vi "Pre-chirper control L1.vi"(7 "State":enum16{"Initialise", "Query", "Close"}(ring), 8 "error in (no error)":errorcluster, 9 "Data to Set":dbl, 10 "Pre-chirper commands":T2, 11 "Visa resource":T1) -> (0 "error out":errorcluster, 3 "number":dbl)   [LabVIEW 2020]
uses:
  Prechirper commands.ctl
  Serial Comms/Visa resource.ctl
  Serial Comms/Serial - Settings.ctl
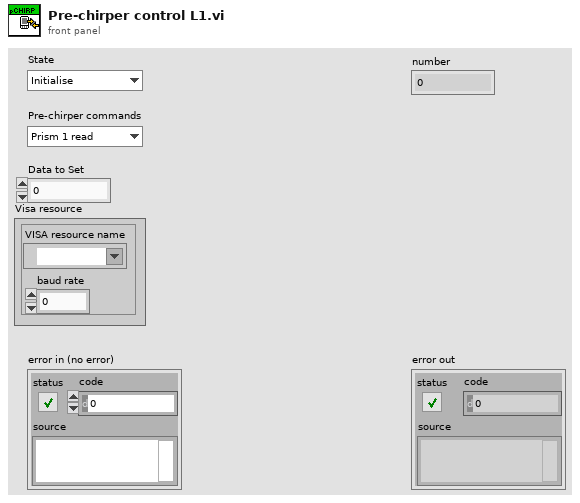
[diagram p1: front panel]
types:
  T1 = typedef "Visa resource.ctl" = cluster{"VISA resource name":refnum<visa-resource-name>, "baud rate":u32}
  T2 = typedef "Prechirper commands.ctl" = enum16{"Prism 1 read", "Prism 1 set", "Prism 2 read", "Prism 2 set", "Wavelength read", "Wavelength Femto set", "Wavelength Femto and Laser set", "GVD curve number read", "GVD curve number set"}
  T3 = typedef "Serial - Settings.ctl" = cluster{"VISA resource name ":refnum<visa-resource-name>, "baud rate":u32, "data bits":u16, "parity":enum16{"None", "Odd", "Even", "Mark", "Space"}, "stop bits":u16, "flow control":u16}
  T4 = enum16{"Initialise", "Read Handle", "Command & Query", "Close"}
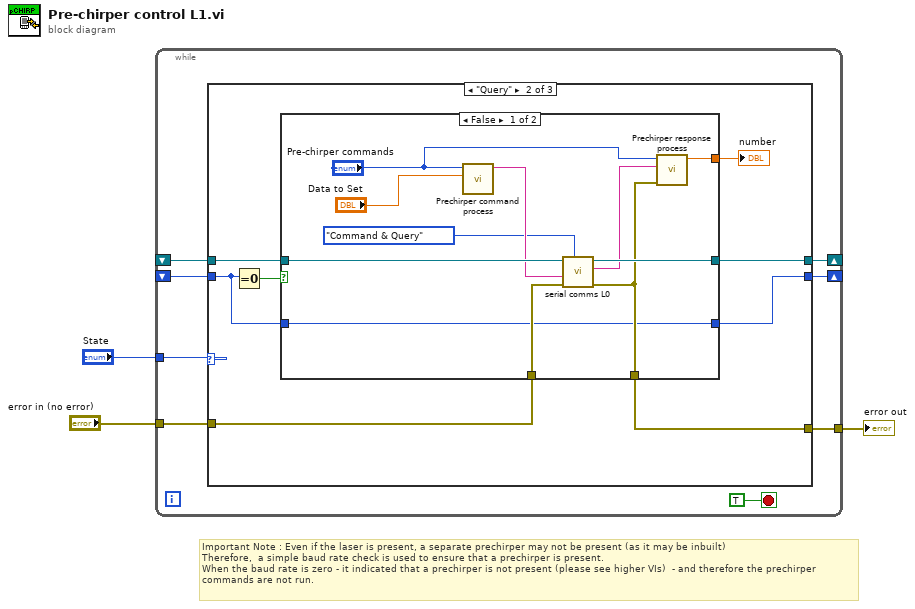
[diagram p0: block diagram]
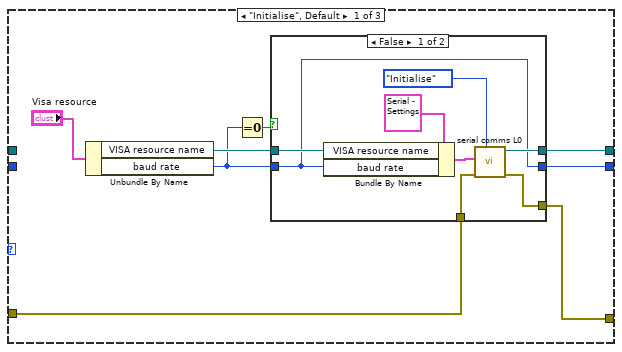
[diagram p2: hidden frame]
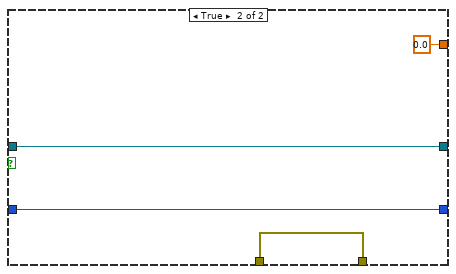
[diagram p4: hidden frame]
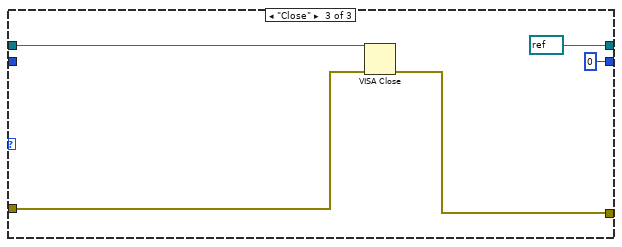
[diagram p5: hidden frame]
diagram:
  # "Important Note : Even if the laser is present, a separate prechirper may not be present (as it may be inbuilt)\nTherefore,  a simple baud rate check is used to ensure that a prechirper is present.\nWhen the baud rate is zero - it indicated that a prechirper is not present (please see higher VIs)  - and therefore the prechirper\ncommands are not run."
  n1 = while {
    tunnel: "State" -> [w10]
    tunnel: "error in (no error)" -> [w9]
    tunnel: [w8] -> w1
    shift-right: [w7] -> _
    shift-left: _ -> [w6]
    shift-right: [w5] -> _
    shift-left: _ -> [w4]
    stop <- TRUE stop-if-true
    n2 = case shown="\"Query\"" w10 {
      tunnel: w9 -> [w19 w38 w57]
      tunnel: [w18 w35 w56] -> w8
      tunnel: [w17 w36 refnum<visa-resource-name> refnum ("VISA resource name out")] -> w7
      tunnel: w6 -> [_ w37 w58]
      tunnel: [w12 w31 u32 0 ("baud rate")] -> w5
      tunnel: w4 -> [_ w32 _]
      frame "Initialise", Default {
        n3 = Unbundle By Name("Visa resource") -> ("VISA resource name"=w15:refnum<visa-resource-name>, "baud rate"=w14:u32)
        n4 = Equal To 0?(x=w14) -> (x = 0?=w13:bool)
        n5 = case shown="False" w13 {
          tunnel: w19 -> [w27 w29]
          tunnel: [w26 w29] -> w18
          tunnel: [w25 w30] -> w17
          tunnel: w15 -> [w22 w30]
          tunnel: w14 -> [w20 w28]
          tunnel: [w20 w28] -> w12
          frame False {
            n6 = Bundle By Name(cluster=T3 {"VISA resource name "="COM12", "baud rate"=115200, "data bits"=8, "parity"=enum."None", "stop bits"=10, "flow control"=0} ("Serial Settings"), "VISA resource name"=w22, "baud rate"=w20) -> (w21:T3)
            n7 = call "serial comms L0.vi"("Comms Control"=T4."Initialise", "error IN"=w27, "Serial Settings"=w21) -> ("Error OUT"=w26:errorcluster, "VISA resource name out"=w25:refnum<visa-resource-name>)  [unwired: 3 in, 4 out]
          }
          frame True {
          }
        }
      }
      frame "Query" {
        n8 = Equal To 0?(x=w32) -> (x = 0?=w33:bool)
        n9 = case shown="False" w33 {
          tunnel: w38 -> [w48 w53]
          tunnel: w37 -> [w47 w52]
          tunnel: [w44 w52] -> w36
          tunnel: [w42 w53] -> w35
          tunnel: [w41 0.0 ("number")] -> w34
          tunnel: [w39 w50] -> w31
          tunnel: w32 -> [w39 w50]
          frame False {
            n10 = call "Prechirper command process.vi"("Data to Set"="Data to Set", "Pre-chirper commands"="Pre-chirper commands") -> ("Comand String"=w46:string)  [unwired: 9 in]
            n11 = call "serial comms L0.vi"("Comms Control"=T4."Command & Query", "error IN"=w48, "Command String"=w46, "VISA resource name"=w47) -> ("Error OUT"=w42:errorcluster, "Response"=w43:string, "VISA resource name out"=w44:refnum<visa-resource-name>)  [unwired: 2 in, 3 out]
            n12 = call "Prechirper response process.vi"("error in (no error)"=w42, "Prechirper response"=w43, "Pre-chirper commands"="Pre-chirper commands") -> ("number"=w41:dbl)  [unwired: 6 in, 2 out]
          }
          frame True {
          }
        }
        "number" <- w34
      }
      frame "Close" {
        n13 = VISA Close(VISA resource name=w58, error in (no error)=w57) -> (error out=w56:errorcluster)
      }
    }
  }
  "error out" <- w1
